vi "四位双向移位寄存器74HC194功能的测试.vi"() -> ()   [LabVIEW 2018]
panel:
  in  "结束":bool
  in  "Dsl":bool
  in  "Dsr":bool
  in  "cp":bool
  in  "CR`":bool
  in  "S1":bool
  in  "S0":bool
  in  "D0":bool
  in  "D1":bool
  in  "D2":bool
  in  "D3":bool
  out "Q0":bool
  out "Q1":bool
  out "Q2":bool
  out "Q3":bool
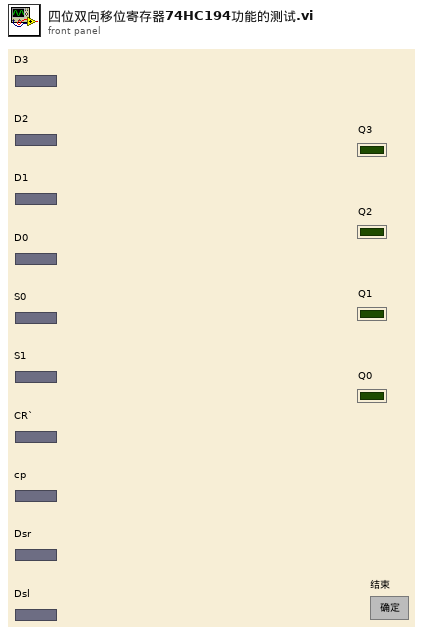
[diagram p1: front panel]
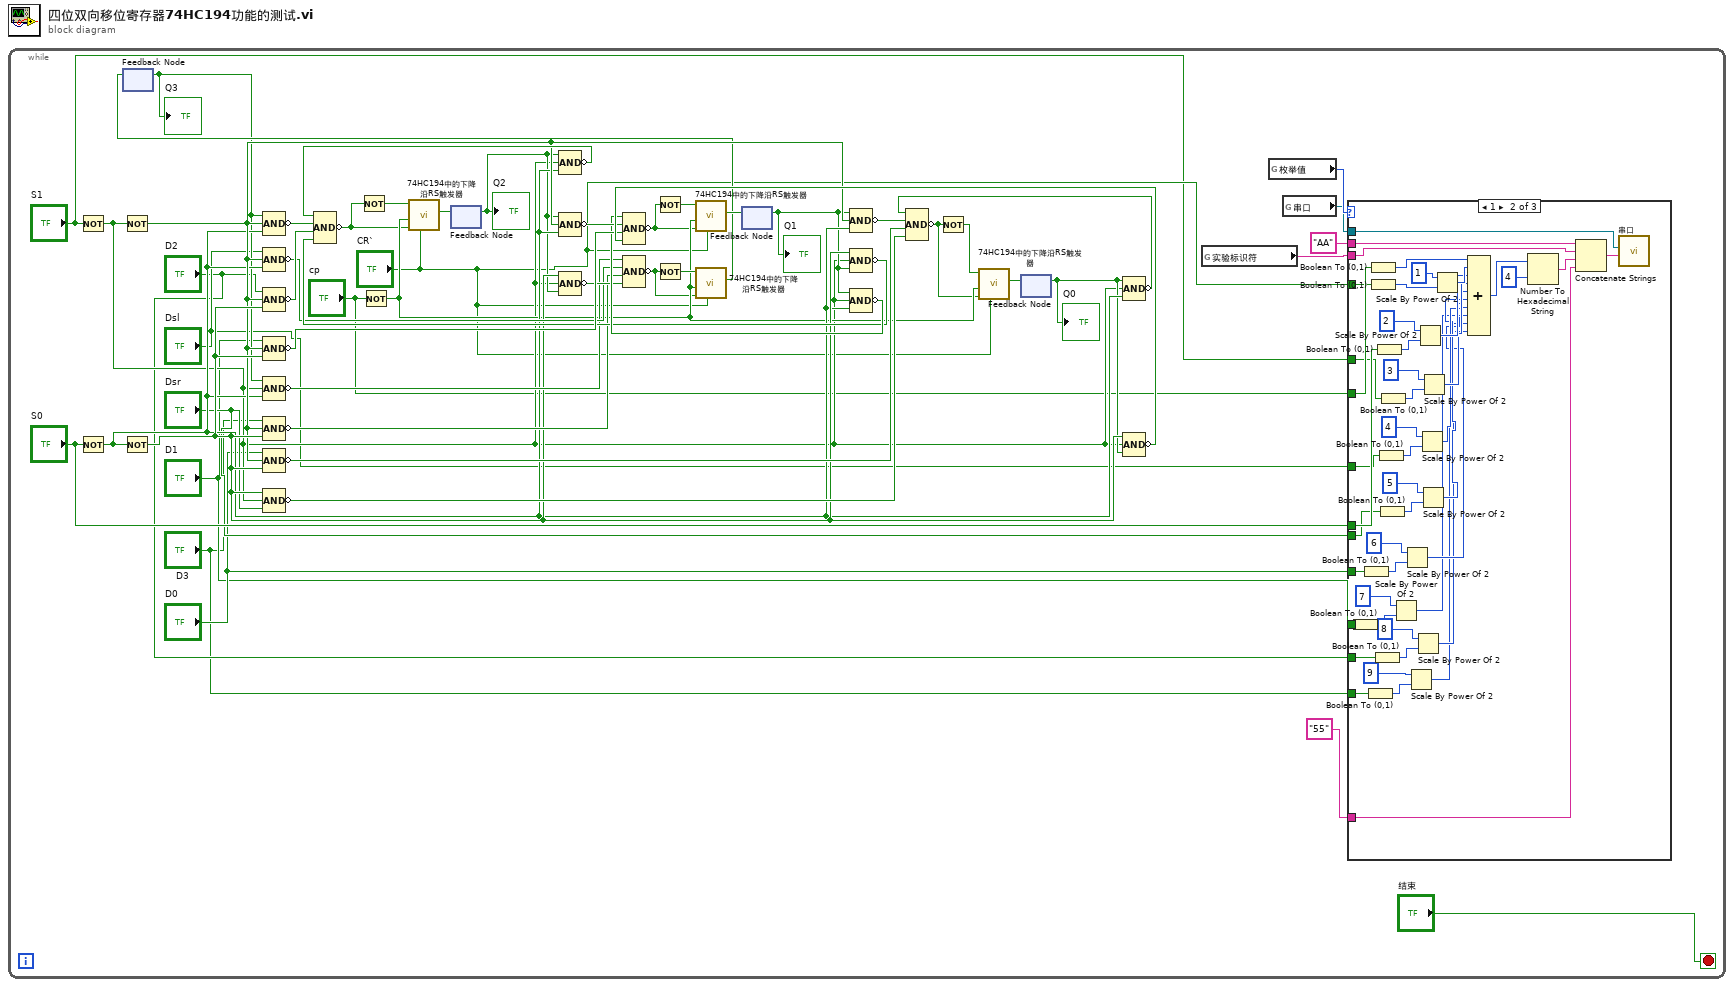
[diagram p0: block diagram]
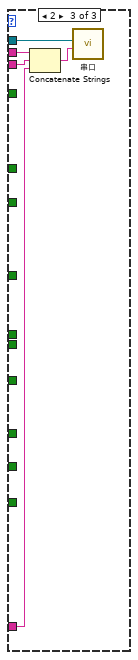
[diagram p3: hidden frame]
diagram:
  n1 = while {
    stop <- "结束" stop-if-true
    n2 = Not(x="S1") -> (.not. x?=w17:bool)
    n3 = Not(x="S0") -> (.not. x?=w35:bool)
    n4 = Not(x=w17) -> (.not. x?=w36:bool)
    n5 = Not(x=w35) -> (.not. x?=w37:bool)
    n6 = feedback #1() -> (w18:bool)  [unwired: 1 in]
    "Q3" <- w18
    n7 = Compound Arithmetic op=AND ("复合运算")(w18, w36, w35) -> (invert w43:bool)
    n8 = Compound Arithmetic op=AND ("复合运算")("Dsl", w36, w35) -> (invert w39:bool)
    n9 = Compound Arithmetic op=AND ("复合运算")("D2", w36, w37) -> (invert w44:bool)
    n10 = Compound Arithmetic op=AND ("复合运算")("D1", w36, w37) -> (invert w48:bool)
    n11 = Compound Arithmetic op=AND ("复合运算")(w18, w17, w35) -> (invert w38:bool)
    n12 = Compound Arithmetic op=AND ("复合运算")("D3", w36, w37) -> (invert w40:bool)
    n13 = Compound Arithmetic op=AND ("复合运算")("D0", w36, w37) -> (invert w52:bool)
    n14 = Compound Arithmetic op=AND ("复合运算")(w37, w17, "Dsr") -> (invert w53:bool)
    n15 = Not(x="cp") -> (.not. x?=w30:bool)
    n16 = feedback #2() -> (w20:bool)  [unwired: 1 in]
    "Q2" <- w20
    n17 = Compound Arithmetic op=AND ("复合运算")(w20, w17, w35) -> (invert w42:bool)
    n18 = Compound Arithmetic op=AND ("复合运算")(w20, w36, w35) -> (invert w47:bool)
    n19 = Compound Arithmetic op=AND ("复合运算")(w37, w17, w20) -> (invert w41:bool)
    n20 = Compound Arithmetic op=AND ("复合运算")(w38, w39, w40, w41) -> (invert w22:bool)
    n21 = Not(x=w22) -> (.not. x?=w32:bool)
    n22 = call "74HC194中的下降沿RS触发器.vi"("R0"="CR`", "R"=w22, "CP"=w30, "S"=w32) -> ("Q"=w19:bool)  [unwired: 7 in]
    n23 = feedback-in #1(w19) -> ()
    n24 = feedback #3() -> (w26:bool)  [unwired: 1 in]
    "Q1" <- w26
    n25 = Compound Arithmetic op=AND ("复合运算")(w26, w36, w35) -> (invert w51:bool)
    n26 = Compound Arithmetic op=AND ("复合运算")(w37, w17, w26) -> (invert w45:bool)
    n27 = Compound Arithmetic op=AND ("复合运算")(w42, w43, w44, w45) -> (invert w23:bool)
    n28 = Not(x=w23) -> (.not. x?=w31:bool)
    n29 = call "74HC194中的下降沿RS触发器.vi"("R0"="CR`", "R"=w23, "CP"=w30, "S"=w31) -> ("Q"=w21:bool)  [unwired: 7 in]
    n30 = feedback-in #2(w21) -> ()
    n31 = Compound Arithmetic op=AND ("复合运算")(w26, w17, w35) -> (invert w46:bool)
    n32 = feedback #4() -> (w28:bool)  [unwired: 1 in]
    "Q0" <- w28
    n33 = Compound Arithmetic op=AND ("复合运算")(w28, w17, w35) -> (invert w50:bool)
    n34 = Compound Arithmetic op=AND ("复合运算")(w50, w51, w52, w53) -> (invert w25:bool)
    n35 = Not(x=w25) -> (.not. x?=w34:bool)
    n36 = call "74HC194中的下降沿RS触发器.vi"("R0"="CR`", "R"=w25, "CP"=w30, "S"=w34) -> ("Q"=w29:bool)  [unwired: 7 in]
    n37 = feedback-in #4(w29) -> ()
    n38 = Compound Arithmetic op=AND ("复合运算")(w37, w17, w28) -> (invert w49:bool)
    n39 = Compound Arithmetic op=AND ("复合运算")(w46, w47, w48, w49) -> (invert w24:bool)
    n40 = Not(x=w24) -> (.not. x?=w33:bool)
    n41 = call "74HC194中的下降沿RS触发器.vi"("R0"="CR`", "R"=w24, "CP"=w30, "S"=w33) -> ("Q"=w27:bool)  [unwired: 7 in]
    n42 = feedback-in #3(w27) -> ()
    n43 = global read "全局变量.vi" "实验标识符"() -> (w13:string)
    n44 = global read "全局变量.vi" "枚举值"() -> (w15:i8)
    n45 = global read "全局变量.vi" "串口"() -> (w14:refnum<visa-resource-name>)
    n46 = case shown="1" w15 {
      tunnel: w14 -> [_ w94 w102]
      tunnel: w13 -> [_ w93 w103]
      tunnel: "55" -> [_ w92 w100]
      tunnel: "AA" -> [_ w91 w101]
      tunnel: "cp" -> [_ w67 _]
      tunnel: "CR`" -> [_ w66 _]
      tunnel: "S0" -> [_ w65 _]
      tunnel: "S1" -> [_ w64 _]
      tunnel: "Dsl" -> [_ w63 _]
      tunnel: "Dsr" -> [_ w62 _]
      tunnel: "D0" -> [_ w61 _]
      tunnel: "D1" -> [_ w60 _]
      tunnel: "D2" -> [_ w59 _]
      tunnel: "D3" -> [_ w58 _]
      frame 0, Default {
      }
      frame 1 {
        n47 = Boolean To (0,1)(Boolean=w60) -> (0, 1=w73:i16)
        n48 = Boolean To (0,1)(Boolean=w61) -> (0, 1=w75:i16)
        n49 = Boolean To (0,1)(Boolean=w58) -> (0, 1=w69:i16)
        n50 = Boolean To (0,1)(Boolean=w67) -> (0, 1=w98:i16)
        n51 = Boolean To (0,1)(Boolean=w66) -> (0, 1=w96:i16)
        n52 = Boolean To (0,1)(Boolean=w59) -> (0, 1=w71:i16)
        n53 = Boolean To (0,1)(Boolean=w65) -> (0, 1=w86:i16)
        n54 = Boolean To (0,1)(Boolean=w63) -> (0, 1=w82:i16)
        n55 = Boolean To (0,1)(Boolean=w62) -> (0, 1=w80:i16)
        n56 = Boolean To (0,1)(Boolean=w64) -> (0, 1=w84:i16)
        n57 = Scale By Power Of 2(n=7, x=w73) -> (x*2^n=w56:i16)
        n58 = Scale By Power Of 2(n=6, x=w75) -> (x*2^n=w57:i16)
        n59 = Scale By Power Of 2(n=9, x=w69) -> (x*2^n=w54:i16)
        n60 = Scale By Power Of 2(n=8, x=w71) -> (x*2^n=w55:i16)
        n61 = Scale By Power Of 2(n=2, x=w86) -> (x*2^n=w87:i16)
        n62 = Scale By Power Of 2(n=4, x=w82) -> (x*2^n=w77:i16)
        n63 = Scale By Power Of 2(n=5, x=w80) -> (x*2^n=w76:i16)
        n64 = Scale By Power Of 2(n=3, x=w84) -> (x*2^n=w78:i16)
        n65 = Scale By Power Of 2(n=1, x=w96) -> (x*2^n=w97:i16)
        n66 = Compound Arithmetic op=ADD ("复合运算")(w98, w97, w87, w78, w77, w76, w57, w56, w55, w54) -> (w90:i16)
        n67 = Number To Hexadecimal String(1:4, 2:w90) -> (0:w88:string)
        n68 = Concatenate Strings(w91, w93, w88, w92) -> (w99:string)
        n69 = call "串口.vi"("字符串"=w99, "VISA resource name"=w94) -> ()  [unwired: 10 in]
      }
      frame 2 {
        n70 = Concatenate Strings(w101, w103, w100) -> (w104:string)
        n71 = call "串口.vi"("字符串"=w104, "VISA resource name"=w102) -> ()  [unwired: 10 in]
      }
    }
  }
